vi "5-5_ Push Counter(LatchWhenReleased).vi"() -> ()   [LabVIEW 2014]
doc: "This example demonstrates how to read one channel of digital input from a LINX device.\n------------------------------------\nAuther: Koji Ohashi\nChanged: Hirotake Watashima\nCopyright (c) 2020 Japan LabVIEW Users Group, Volunteer members.\nThis VI is released under the MIT License.\nhttp://opensource.org/licenses/mit-license.php\n------------------------------------"
uses:
  <vilib>/MakerHub/LINX/LMH-LINX.lvlib
  <vilib>/MakerHub/LINX/Public/Utilities/Open Serial.vi
  <vilib>/MakerHub/LINX/Public/Peripherals/Digital/Digital Read 1 Chan.vi
panel:
  in  "Serial Port":refnum<visa-resource-name>
  out "Count":u32
  out "DI Value":bool
  in  "DI Channel":u8=8
  in  "Stop Button":bool
  # "LINX Device Settings"
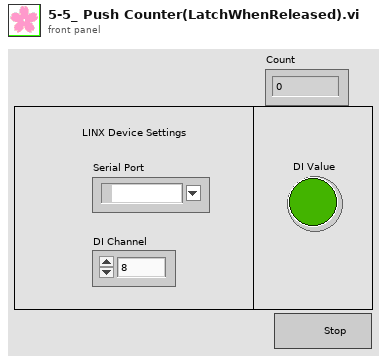
[diagram p1: front panel]
types:
  T1 = typedef "LMH-LINX.lvlib/LINX Ref.ctl" = cluster{"IO":T2, "Interface":T3, "LINX Device Config":T4}
  T2 = typedef "LMH-LINX.lvlib/Platform.ctl" = enum16{"Remote", "Local"}
  T3 = typedef "LMH-LINX.lvlib/Interface.ctl" = enum16{"Serial", "TCP"}
  T4 = typedef "LMH-LINX.lvlib/Device.lvlib/LINX Device Config.ctl" = cluster{"Interface":T3, "COM Port":refnum<visa-resource-name>, "TCP Configuration":T5, "Device Family":u8, "Device ID":u8, "Device Name":string, "TCP Ref":refnum<k5>, "Channels":T6}
  T5 = typedef "LMH-LINX.lvlib/Device.lvlib/TCP Config.ctl" = cluster{"IP Address":string, "Port":u16}
  T6 = typedef "LMH-LINX.lvlib/Channels.ctl" = cluster{"DI":u8[], "DO":u8[], "AI":u8[], "AO":u8[], "PWM":u8[], "QE":u8[], "UART":u8[], "I2C 2":u8[], "SPI":u8[], "CAN":u8[], "Servo":u8[], "AI Ref (V)":dbl, "AI Resolution (Bits)":u8, "AO Ref (V)":dbl, "AO Resolution (Bits)":u8}
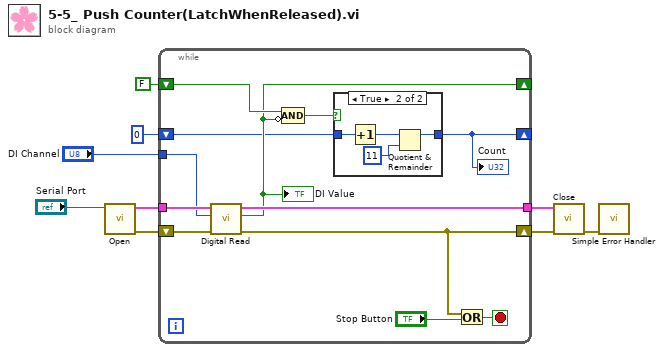
[diagram p0: block diagram]
diagram:
  n1 = call-poly <vilib>:"Open.vi"("Serial Port"="Serial Port") -> ("Error Out"=w8:errorcluster, "LINX Resource"=w9:T1)  [unwired: 8 in, 1 out]
  n2 = while {
    tunnel: w9 -> [w17]
    tunnel: [w18] -> w7
    shift-right: [w19] -> w6
    shift-left: w8 -> [w16]
    tunnel: "DI Channel" -> [w15]
    shift-right: [w13] -> _
    shift-left: FALSE ("DI Value") -> [w14]
    shift-right: [w10] -> _
    shift-left: u32 0 -> [w11]
    stop <- w21 stop-if-true
    n3 = call-poly <vilib>:"Digital Read.vi"("Error In"=w16, "DI Channel"=w15, "LINX Resource"=w17) -> ("Error Out"=w19:errorcluster, "DI Value"=w13:bool, "LINX Resource"=w18:T1)  [unwired: 6 in]
    "DI Value" <- w13
    n4 = Compound Arithmetic op=AND ("複合演算")(w14, invert w13) -> (w12:bool)
    n5 = case shown="TRUE" w12 {
      tunnel: w11 -> [w22 w25]
      tunnel: [w22 w23] -> w10
      frame False {
      }
      frame True {
        n6 = Increment(x=w25) -> (x+1=w24:u32)
        n7 = Quotient & Remainder(x=w24, y=u32 11) -> (x-y*floor(x/y)=w23:u32)  [unwired: 1 out]
      }
    }
    "Count" <- w10
    n8 = Or(x=w19, y="Stop Button") -> (x .or. y?=w21:bool)
  }
  n9 = call <vilib>:"Close.vi"("Error In"=w6, "LINX Resource"=w7) -> ("Error Out"=w5:errorcluster)  [unwired: 9 in]
  n10 = call <vilib>:"Simple Error Handler.vi"("error in (no error)"=w5) -> ()  [unwired: 4 in, 5 out]
